vi "Visa_Reset_Clear.vi"(0 "VISA resource name":refnum<visa-resource-name>="GPIB0::18::INSTR", 1 "Send *CLS":bool, 2 "Restore Defaults":bool, 3 "Close VISA session":bool, 11 "error in (no error)":errorcluster, 14 "Send *RST":bool=TRUE) -> (4 "VISA resource name Out":refnum<visa-resource-name>, 15 "error out":errorcluster)   [LabVIEW 2018]
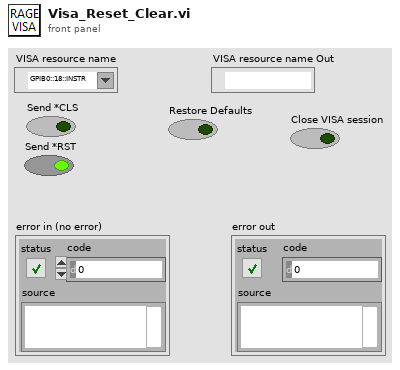
[diagram p1: front panel]
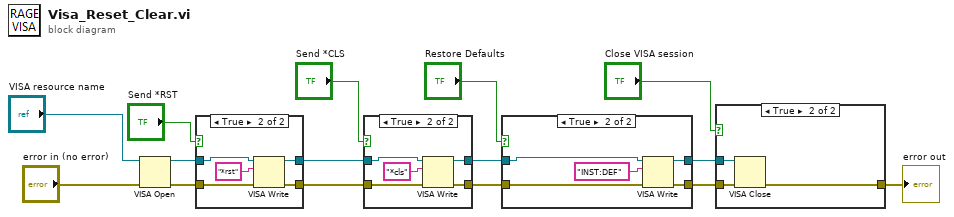
[diagram p0: block diagram]
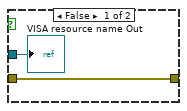
[diagram p3: hidden frame]
diagram:
  n1 = VISA Open(error in (no error)="error in (no error)", VISA resource name="VISA resource name") -> (VISA resource name=w14:refnum<visa-resource-name>, error out=w12:errorcluster)  [unwired: 3 in]
  n2 = case shown="True" "Send *RST" {
    tunnel: [w16 w22] -> w15
    tunnel: w14 -> [w16 w21]
    tunnel: w12 -> [w17 w19]
    tunnel: [w17 w18] -> w9
    frame False {
    }
    frame True {
      n3 = VISA Write(VISA resource name=w21, write buffer="*rst", error in (no error)=w19) -> (VISA resource name out=w22:refnum<visa-resource-name>, error out=w18:errorcluster)  [unwired: 1 out]
    }
  }
  n4 = case shown="True" "Send *CLS" {
    tunnel: w15 -> [w24 w29]
    tunnel: [w24 w28] -> w4
    tunnel: w9 -> [w23 w26]
    tunnel: [w23 w25] -> w5
    frame False {
    }
    frame True {
      n5 = VISA Write(VISA resource name=w29, write buffer="*cls", error in (no error)=w26) -> (VISA resource name out=w28:refnum<visa-resource-name>, error out=w25:errorcluster)  [unwired: 1 out]
    }
  }
  n6 = case shown="True" "Restore Defaults" {
    tunnel: w4 -> [w31 w36]
    tunnel: [w31 w35] -> w3
    tunnel: w5 -> [w30 w33]
    tunnel: [w30 w32] -> w2
    frame False {
    }
    frame True {
      n7 = VISA Write(VISA resource name=w36, write buffer="INST:DEF", error in (no error)=w33) -> (VISA resource name out=w35:refnum<visa-resource-name>, error out=w32:errorcluster)  [unwired: 1 out]
    }
  }
  n8 = case shown="True" "Close VISA session" {
    tunnel: [w38 w41] -> w11
    tunnel: w3 -> [w37 w40]
    tunnel: w2 -> [w38 w39]
    frame False {
      "VISA resource name Out" <- w37
    }
    frame True {
      n9 = VISA Close(VISA resource name=w40, error in (no error)=w39) -> (error out=w41:errorcluster)
    }
  }
  "error out" <- w11
